vi "FeaturesCalculation.vi"(0 "bw":T1(plugin-control)) -> (2 "PP":dbl, 3 "top":i32, 4 "FDIC":sgl, 5 "PAR":dbl, 6 "PW":dbl, 7 "MPH":dbl, 8 "TPA":dbl, 9 "FDNIC":sgl, 10 "TBR":dbl)   [LabVIEW 2015]
uses:
  <vilib>/vision/NI_Vision_Development_Module.lvlib
  Realse/fractaldim.dll
panel:
  out "bw 2":T1(plugin-control)
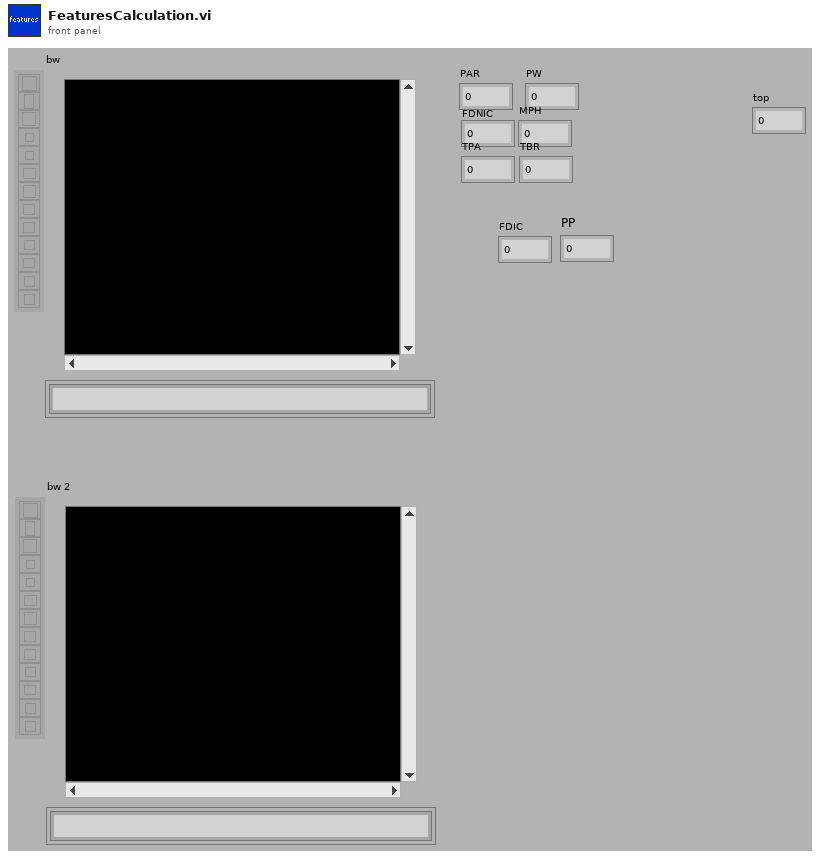
[diagram p1: front panel]
types:
  T1 = typedef "IMAQ Image.ctl" = refnum<image>
  T2 = typedef "Particle Parameters" = i32
  T3 = typedef "Image Type" = u32
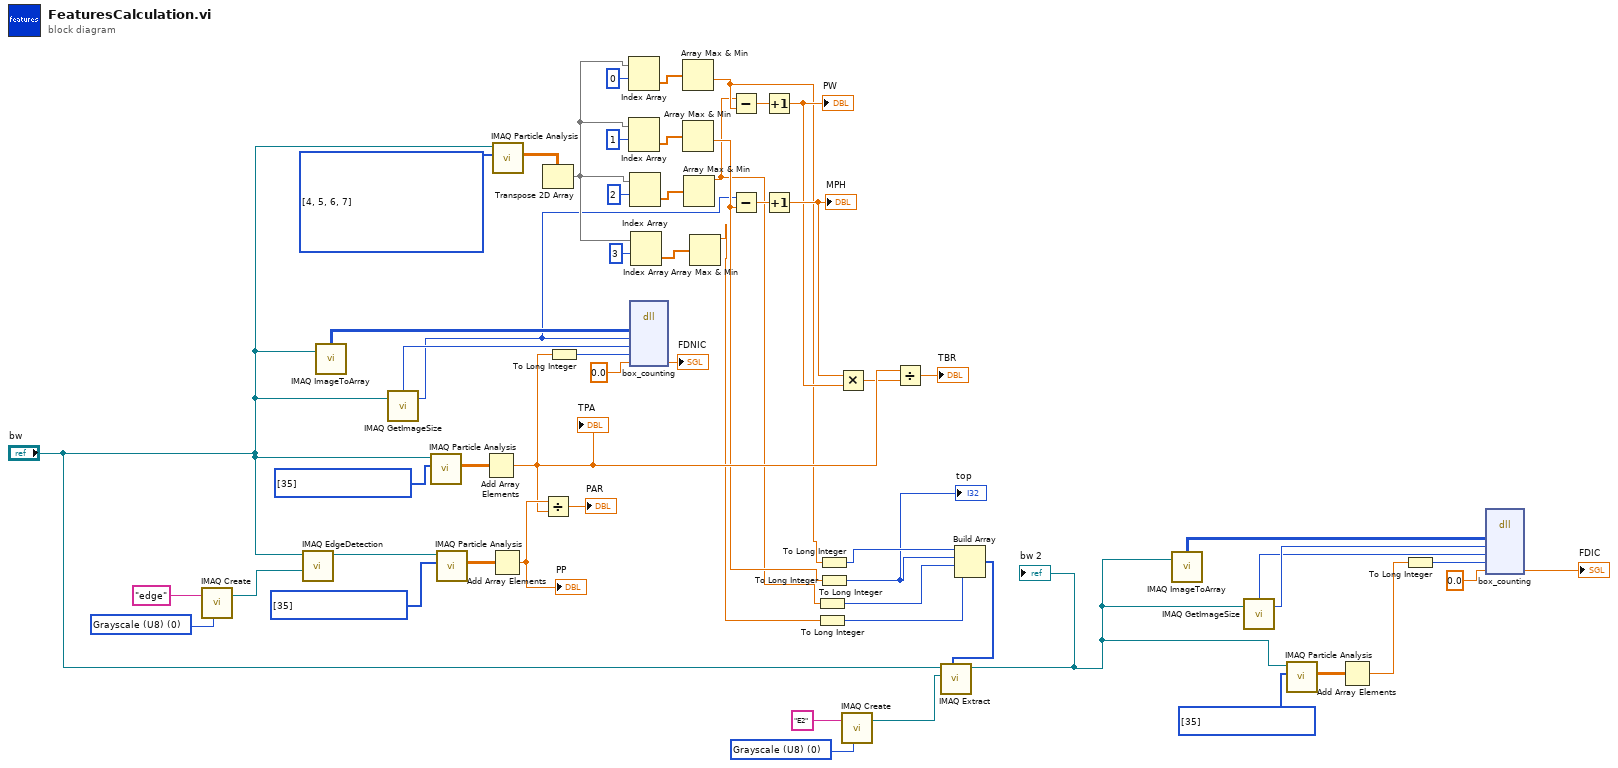
[diagram p0: block diagram]
diagram:
  w4 = T2[] [35] items=["Center of Mass X", "Center of Mass Y", "First Pixel X", "First Pixel Y", "Bounding Rect Left", "Bounding Rect Top", "Bounding Rect Right", "Bounding Rect Bottom", "Max Feret Diameter Start X", "Max Feret Diameter Start Y", "Max Feret Diameter End X", "Max Feret Diameter End Y", "Max Horiz. Segment Length Left", "Max Horiz. Segment Length Right", "Max Horiz. Segment Length Row", "-", "Bounding Rect Width", "Bounding Rect Height", "Bounding Rect Diagonal", "Perimeter", "Convex Hull Perimeter", "Holes' Perimeter", "Max Feret Diameter", "Equivalent Ellipse Major Axis", "Equivalent Ellipse Minor Axis", "Equivalent Ellipse Minor Axis (Feret)", "Equivalent Rect Long Side", "Equivalent Rect Short Side", "Equivalent Rect Diagonal", "Equivalent Rect Short Side (Feret)", "Average Horiz. Segment Length", "Average Vert. Segment Length", "Hydraulic Radius", "Waddel Disk Diameter", "-", "Area", "Holes' Area", "Particle & Holes' Area", "Convex Hull Area", "Image Area", "-", "Number of Holes", "Number of Horiz. Segments", "Number of Vert. Segments", "-", "Orientation", "Max Feret Diameter Orientation", "-", "% Area/Image Area", "% Area/(Particle & Holes' Area)", "Ratio of Equivalent Ellipse Axes", "Ratio of Equivalent Rect Sides", "-", "Elongation Factor", "Compactness Factor", "Heywood Circularity Factor", "Type Factor", "-", "Sum X", "Sum Y", "Sum XX", "Sum XY", "Sum YY", "Sum XXX", "Sum XXY", "Sum XYY", "Sum YYY", "-", "Moment of Inertia XX", "Moment of Inertia XY", "Moment of Inertia YY", "Moment of Inertia XXX", "Moment of Inertia XXY", "Moment of Inertia XYY", "Moment of Inertia YYY", "Norm. Moment of Inertia XX", "Norm. Moment of Inertia XY", "Norm. Moment of Inertia YY", "Norm. Moment of Inertia XXX", "Norm. Moment of Inertia XXY", "Norm. Moment of Inertia XYY", "Norm. Moment of Inertia YYY", "Hu Moment 1", "Hu Moment 2", "Hu Moment 3", "Hu Moment 4", "Hu Moment 5", "Hu Moment 6", "Hu Moment 7"] ("Pixel Measurements")
  w23 = T3 0 items=["Grayscale (U8)", "Grayscale (I16)", "Grayscale (SGL)", "Complex (CSG)", "RGB (U32)", "HSL (U32)", "RGB (U64)", "Grayscale (U16)"] ("Image Type")
  w42 = T2[] [4, 5, 6, 7] items=["Center of Mass X", "Center of Mass Y", "First Pixel X", "First Pixel Y", "Bounding Rect Left", "Bounding Rect Top", "Bounding Rect Right", "Bounding Rect Bottom", "Max Feret Diameter Start X", "Max Feret Diameter Start Y", "Max Feret Diameter End X", "Max Feret Diameter End Y", "Max Horiz. Segment Length Left", "Max Horiz. Segment Length Right", "Max Horiz. Segment Length Row", "-", "Bounding Rect Width", "Bounding Rect Height", "Bounding Rect Diagonal", "Perimeter", "Convex Hull Perimeter", "Holes' Perimeter", "Max Feret Diameter", "Equivalent Ellipse Major Axis", "Equivalent Ellipse Minor Axis", "Equivalent Ellipse Minor Axis (Feret)", "Equivalent Rect Long Side", "Equivalent Rect Short Side", "Equivalent Rect Diagonal", "Equivalent Rect Short Side (Feret)", "Average Horiz. Segment Length", "Average Vert. Segment Length", "Hydraulic Radius", "Waddel Disk Diameter", "-", "Area", "Holes' Area", "Particle & Holes' Area", "Convex Hull Area", "Image Area", "-", "Number of Holes", "Number of Horiz. Segments", "Number of Vert. Segments", "-", "Orientation", "Max Feret Diameter Orientation", "-", "% Area/Image Area", "% Area/(Particle & Holes' Area)", "Ratio of Equivalent Ellipse Axes", "Ratio of Equivalent Rect Sides", "-", "Elongation Factor", "Compactness Factor", "Heywood Circularity Factor", "Type Factor", "-", "Sum X", "Sum Y", "Sum XX", "Sum XY", "Sum YY", "Sum XXX", "Sum XXY", "Sum XYY", "Sum YYY", "-", "Moment of Inertia XX", "Moment of Inertia XY", "Moment of Inertia YY", "Moment of Inertia XXX", "Moment of Inertia XXY", "Moment of Inertia XYY", "Moment of Inertia YYY", "Norm. Moment of Inertia XX", "Norm. Moment of Inertia XY", "Norm. Moment of Inertia YY", "Norm. Moment of Inertia XXX", "Norm. Moment of Inertia XXY", "Norm. Moment of Inertia XYY", "Norm. Moment of Inertia YYY", "Hu Moment 1", "Hu Moment 2", "Hu Moment 3", "Hu Moment 4", "Hu Moment 5", "Hu Moment 6", "Hu Moment 7"] ("Pixel Measurements")
  w50 = T2[] [35] items=["Center of Mass X", "Center of Mass Y", "First Pixel X", "First Pixel Y", "Bounding Rect Left", "Bounding Rect Top", "Bounding Rect Right", "Bounding Rect Bottom", "Max Feret Diameter Start X", "Max Feret Diameter Start Y", "Max Feret Diameter End X", "Max Feret Diameter End Y", "Max Horiz. Segment Length Left", "Max Horiz. Segment Length Right", "Max Horiz. Segment Length Row", "-", "Bounding Rect Width", "Bounding Rect Height", "Bounding Rect Diagonal", "Perimeter", "Convex Hull Perimeter", "Holes' Perimeter", "Max Feret Diameter", "Equivalent Ellipse Major Axis", "Equivalent Ellipse Minor Axis", "Equivalent Ellipse Minor Axis (Feret)", "Equivalent Rect Long Side", "Equivalent Rect Short Side", "Equivalent Rect Diagonal", "Equivalent Rect Short Side (Feret)", "Average Horiz. Segment Length", "Average Vert. Segment Length", "Hydraulic Radius", "Waddel Disk Diameter", "-", "Area", "Holes' Area", "Particle & Holes' Area", "Convex Hull Area", "Image Area", "-", "Number of Holes", "Number of Horiz. Segments", "Number of Vert. Segments", "-", "Orientation", "Max Feret Diameter Orientation", "-", "% Area/Image Area", "% Area/(Particle & Holes' Area)", "Ratio of Equivalent Ellipse Axes", "Ratio of Equivalent Rect Sides", "-", "Elongation Factor", "Compactness Factor", "Heywood Circularity Factor", "Type Factor", "-", "Sum X", "Sum Y", "Sum XX", "Sum XY", "Sum YY", "Sum XXX", "Sum XXY", "Sum XYY", "Sum YYY", "-", "Moment of Inertia XX", "Moment of Inertia XY", "Moment of Inertia YY", "Moment of Inertia XXX", "Moment of Inertia XXY", "Moment of Inertia XYY", "Moment of Inertia YYY", "Norm. Moment of Inertia XX", "Norm. Moment of Inertia XY", "Norm. Moment of Inertia YY", "Norm. Moment of Inertia XXX", "Norm. Moment of Inertia XXY", "Norm. Moment of Inertia XYY", "Norm. Moment of Inertia YYY", "Hu Moment 1", "Hu Moment 2", "Hu Moment 3", "Hu Moment 4", "Hu Moment 5", "Hu Moment 6", "Hu Moment 7"] ("Pixel Measurements")
  w53 = T3 0 items=["Grayscale (U8)", "Grayscale (I16)", "Grayscale (SGL)", "Complex (CSG)", "RGB (U32)", "HSL (U32)", "RGB (U64)", "Grayscale (U16)"] ("Image Type")
  w56 = T2[] [35] items=["Center of Mass X", "Center of Mass Y", "First Pixel X", "First Pixel Y", "Bounding Rect Left", "Bounding Rect Top", "Bounding Rect Right", "Bounding Rect Bottom", "Max Feret Diameter Start X", "Max Feret Diameter Start Y", "Max Feret Diameter End X", "Max Feret Diameter End Y", "Max Horiz. Segment Length Left", "Max Horiz. Segment Length Right", "Max Horiz. Segment Length Row", "-", "Bounding Rect Width", "Bounding Rect Height", "Bounding Rect Diagonal", "Perimeter", "Convex Hull Perimeter", "Holes' Perimeter", "Max Feret Diameter", "Equivalent Ellipse Major Axis", "Equivalent Ellipse Minor Axis", "Equivalent Ellipse Minor Axis (Feret)", "Equivalent Rect Long Side", "Equivalent Rect Short Side", "Equivalent Rect Diagonal", "Equivalent Rect Short Side (Feret)", "Average Horiz. Segment Length", "Average Vert. Segment Length", "Hydraulic Radius", "Waddel Disk Diameter", "-", "Area", "Holes' Area", "Particle & Holes' Area", "Convex Hull Area", "Image Area", "-", "Number of Holes", "Number of Horiz. Segments", "Number of Vert. Segments", "-", "Orientation", "Max Feret Diameter Orientation", "-", "% Area/Image Area", "% Area/(Particle & Holes' Area)", "Ratio of Equivalent Ellipse Axes", "Ratio of Equivalent Rect Sides", "-", "Elongation Factor", "Compactness Factor", "Heywood Circularity Factor", "Type Factor", "-", "Sum X", "Sum Y", "Sum XX", "Sum XY", "Sum YY", "Sum XXX", "Sum XXY", "Sum XYY", "Sum YYY", "-", "Moment of Inertia XX", "Moment of Inertia XY", "Moment of Inertia YY", "Moment of Inertia XXX", "Moment of Inertia XXY", "Moment of Inertia XYY", "Moment of Inertia YYY", "Norm. Moment of Inertia XX", "Norm. Moment of Inertia XY", "Norm. Moment of Inertia YY", "Norm. Moment of Inertia XXX", "Norm. Moment of Inertia XXY", "Norm. Moment of Inertia XYY", "Norm. Moment of Inertia YYY", "Hu Moment 1", "Hu Moment 2", "Hu Moment 3", "Hu Moment 4", "Hu Moment 5", "Hu Moment 6", "Hu Moment 7"] ("Pixel Measurements")
  n1 = call "IMAQ Create"("Image Name"="edge", "Image Type"=w53) -> ("New Image"=w52:T1)  [unwired: 2 in, 2 out]
  n2 = call "IMAQ EdgeDetection"("Image Dst"=w52, "Image Src"="bw") -> ("Image Dst Out"=w55:T1)  [unwired: 4 in, 5 out]
  n3 = call "IMAQ ImageToArray"("Image"="bw") -> ("Image Pixels (U8)"=w46:u8[][])  [unwired: 2 in, 5 out]
  n4 = call "IMAQ GetImageSize"("Image"="bw") -> ("Y Resolution"=w1:i32, "X Resolution"=w43:i32)  [unwired: 1 in, 3 out]
  n5 = call "IMAQ Particle Analysis"("Pixel Measurements"=w50, "Image"="bw") -> ("Particle Measurements (Pixels)"=w51:dbl[][])  [unwired: 3 in, 6 out]
  n6 = call "IMAQ Particle Analysis"("Pixel Measurements"=w56, "Image"=w55) -> ("Particle Measurements (Pixels)"=w57:dbl[][])  [unwired: 3 in, 6 out]
  n7 = Add Array Elements(numeric array=w51) -> (sum=w29:dbl)
  "TPA" <- w29
  n8 = Add Array Elements(numeric array=w57) -> (sum=w49:dbl)
  "PP" <- w49
  n9 = call "IMAQ Particle Analysis"("Pixel Measurements"=w42, "Image"="bw") -> ("Particle Measurements (Pixels)"=w41:dbl[][])  [unwired: 3 in, 6 out]
  n10 = Transpose 2D Array(2D array=w41) -> (transposed array=w32:dbl[][])
  n11 = Divide(x=w49, y=w29) -> (x/y=→"PAR":dbl)
  n12 = To Long Integer(number=w29) -> (32bit integer=w45:i32)
  n13 = Index Array(array=w32, index (row)=0) -> (element=w34:dbl[])  [unwired: 1 in]
  n14 = Index Array(array=w32, index (row)=1) -> (element=w35:dbl[])  [unwired: 1 in]
  n15 = Index Array(array=w32, index (row)=2) -> (element=w39:dbl[])  [unwired: 1 in]
  n16 = dll-call lib="PTH2gabs E文章投稿&51. 代明球老师-玉米胁迫实验\tRGB程序maizeRealsefractaldim.dll" fn="box_counting"("bw"=w46, "row"=w1, "col"=w43, "area"=w45, "FD"=sgl 0.0) -> ("FD"=→"FDNIC":sgl)  [unwired: 7 in, 3 out]
  n17 = Index Array(array=w32, index (row)=3) -> (element=w38:dbl[])  [unwired: 1 in]
  n18 = Array Max & Min(array=w34) -> (min value=w20:dbl)  [unwired: 3 out]
  n19 = Array Max & Min(array=w35) -> (min value=w18:dbl)  [unwired: 3 out]
  n20 = Array Max & Min(array=w39) -> (max value=w16:dbl)  [unwired: 3 out]
  n21 = Array Max & Min(array=w38) -> (max value=w14:dbl)  [unwired: 3 out]
  n22 = Subtract(x=w16, y=w20) -> (x-y=w31:dbl)
  n23 = Subtract(x=w1, y=w18) -> (x-y=w30:dbl)
  n24 = Increment(x=w31) -> (x+1=w26:dbl)
  "PW" <- w26
  n25 = Increment(x=w30) -> (x+1=w27:dbl)
  "MPH" <- w27
  n26 = To Long Integer(number=w16) -> (32bit integer=w15:i32)
  n27 = To Long Integer(number=w14) -> (32bit integer=w13:i32)
  n28 = To Long Integer(number=w20) -> (32bit integer=w19:i32)
  n29 = To Long Integer(number=w18) -> (32bit integer=w17:i32)
  "top" <- w17
  n30 = Multiply(x=w27, y=w26) -> (x*y=w28:dbl)
  n31 = call "IMAQ Create"("Image Name"="E2", "Image Type"=w23) -> ("New Image"=w21:T1)  [unwired: 2 in, 2 out]
  n32 = Divide(x=w29, y=w28) -> (x/y=→"TBR":dbl)
  n33 = Build Array(w19, w17, w15, w13) -> (w12:i32[])
  n34 = call "IMAQ Extract"("Optional Rectangle"=w12, "Image Dst"=w21, "Image Src"="bw") -> ("Image Dst Out"=w2:T1)  [unwired: 3 in, 5 out]
  "bw 2" <- w2
  n35 = call "IMAQ ImageToArray"("Image"=w2) -> ("Image Pixels (U8)"=w6:u8[][])  [unwired: 2 in, 5 out]
  n36 = call "IMAQ GetImageSize"("Image"=w2) -> ("Y Resolution"=w10:i32, "X Resolution"=w9:i32)  [unwired: 1 in, 3 out]
  n37 = call "IMAQ Particle Analysis"("Pixel Measurements"=w4, "Image"=w2) -> ("Particle Measurements (Pixels)"=w3:dbl[][])  [unwired: 3 in, 6 out]
  n38 = Add Array Elements(numeric array=w3) -> (sum=w11:dbl)
  n39 = To Long Integer(number=w11) -> (32bit integer=w7:i32)
  n40 = dll-call lib="PTH2gabs E文章投稿&51. 代明球老师-玉米胁迫实验\tRGB程序maizeRealsefractaldim.dll" fn="box_counting"("bw"=w6, "row"=w10, "col"=w9, "area"=w7, "FD"=sgl 0.0) -> ("FD"=→"FDIC":sgl)  [unwired: 7 in, 3 out]
